vi "Update Weather Display Objects.vi"(8 "Error In":errorcluster, 11 "Display Manager In":refnum<class "Display Manager.lvclass">) -> (0 "Error Out":errorcluster, 3 "Display Manager Out":refnum<class "Display Manager.lvclass">)   [LabVIEW 2019, in "Display Manager.lvclass"]
uses:
  Display Manager.lvclass
  <vilib>/Memosfet/myRIO-Neopixel/RT/String/String.lvclass
  Accessors/Display/Get Display.vi
  <vilib>/Memosfet/myRIO-Neopixel/RT/Display/Display.lvclass
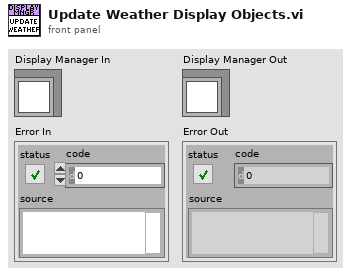
[diagram p1: front panel]
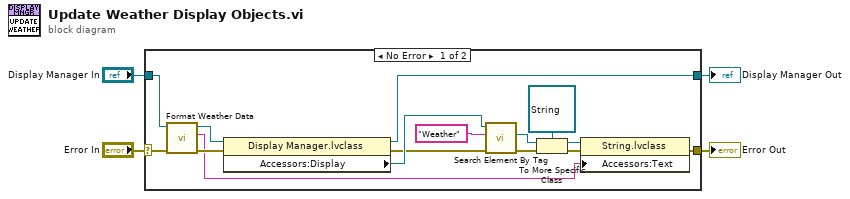
[diagram p0: block diagram]
diagram:
  n1 = case shown="No Error" "Error In" {
    selector: "Error In" -> [w9 w21]
    tunnel: [w19 w21] -> w3
    tunnel: "Display Manager In" -> [w11 w20]
    tunnel: [w6 w20] -> w1
    frame No Error {
      n2 = call "Format Weather Data.vi"("Error In"=w9, "Display Manager In"=w11) -> ("Error Out"=w8:errorcluster, "Weather String"=w7:string, "Display Manager Out"=w10:refnum<class "Display Manager.lvclass">)  [unwired: 7 in]
      n3 = property class="Display Manager.lvclass"(reference=w10, error in=w8) -> (reference out=w6:refnum<class "Display Manager.lvclass">, error out=w5:errorcluster, "Accessors:Display"=w13:refnum<class "Display.lvclass">)
      n4 = call <vilib>:"Search Element By Tag.vi"("Error In"=w5, "Element Tag"="Weather" ("Tag"), "Display In"=w13) -> ("Error Out"=w14:errorcluster, "Display Element"=w15:refnum<class "Display Element.lvclass">)  [unwired: 5 in, 2 out]
      n5 = To More Specific Class(target class=refnum<class "String.lvclass"> refnum ("Pixel In"), reference=w15, error in=w14) -> (specific class reference=w17:refnum<class "String.lvclass">, error out=w16:errorcluster)
      n6 = property class="String.lvclass"(reference=w17, error in=w16, "Accessors:Text"=w7) -> (error out=w19:errorcluster)  [unwired: 1 out]
    }
    frame Error {
    }
  }
  "Display Manager Out" <- w1
  "Error Out" <- w3
